vi "GV-PlotRscaleIndicator.vi"(4 "Format":string, 5 "ActualValues":dbl[](array[numeric]), 6 "type":enum16{"background", "foreground"}(ring), 7 "Graph-ref":refnum<vi>, 8 "error in (no error)":errorcluster, 9 "SelProperties":T1[](array[typedef]), 10 "Plot":i32, 11 "Picture IN":picture) -> (0 "error out":errorcluster, 3 "Picture OUT":picture)   [LabVIEW 2020, in "Sgraph_lib_V1.lvlib" / "Gviewer.lvclass"]
doc: "Andre Koelewijn, 17 feb 2022\n\nPlot an indicator on the Right side of the Graph"
uses:
  Gviewer.lvclass
  controls/Typedef_SelProperties.ctl
  controls/Typedef_LineType.ctl
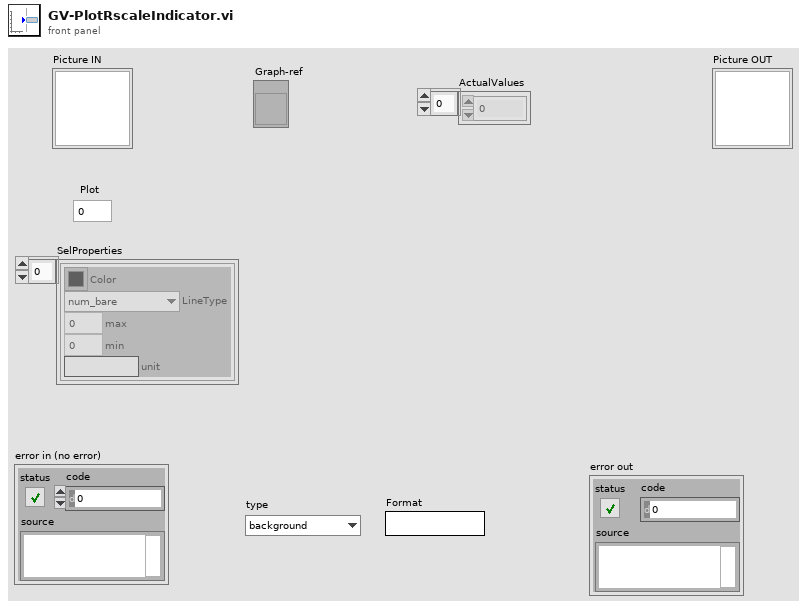
[diagram p1: front panel]
types:
  T1 = typedef "Sgraph_lib_V1.lvlib/Gviewer.lvclass/Typedef_SelProperties.ctl" = cluster{"Color":u32, "LineType":T2, "max":dbl, "min":dbl, "unit":string}
  T2 = typedef "Sgraph_lib_V1.lvlib/Gviewer.lvclass/Typedef_LineType.ctl" = enum16{"num_bare", "num_MinMax_Area", "num_MinMax_Lines", "num_MinMax_Forfor", "num_Max_Area", "num_Max_Line", "num_Max_Forfor", "num_Min_Area", "num_Min_Line", "num_Min_Fosfor", "Boolean_Line_01", "Boolean_Area_01", "Boolean_Fosfor_01", "Boolean_Line_TF", "Boolean_Area_TF", "Boolean_Fosfor_TF", "Boolean_OnOff_Line", "Boolean_OnOff_Area", "Boolean_OnOff_Fosfor", "Boolean_spare", "StringEvent_Line", "StringEvent_TimeLine"}
  T3 = cluster{"horizontal":enum16{"left", "center", "right"}, "vertical":enum16{"top", "center", "bottom"}}
  T4 = typedef "LVRectTypeDef.ctl" = cluster{"Left":i16, "Top":i16, "Right":i16, "Bottom":i16}
  T5 = typedef "LVPoint32TypeDef.ctl" = cluster{"Horizontal":i32, "Vertical":i32}
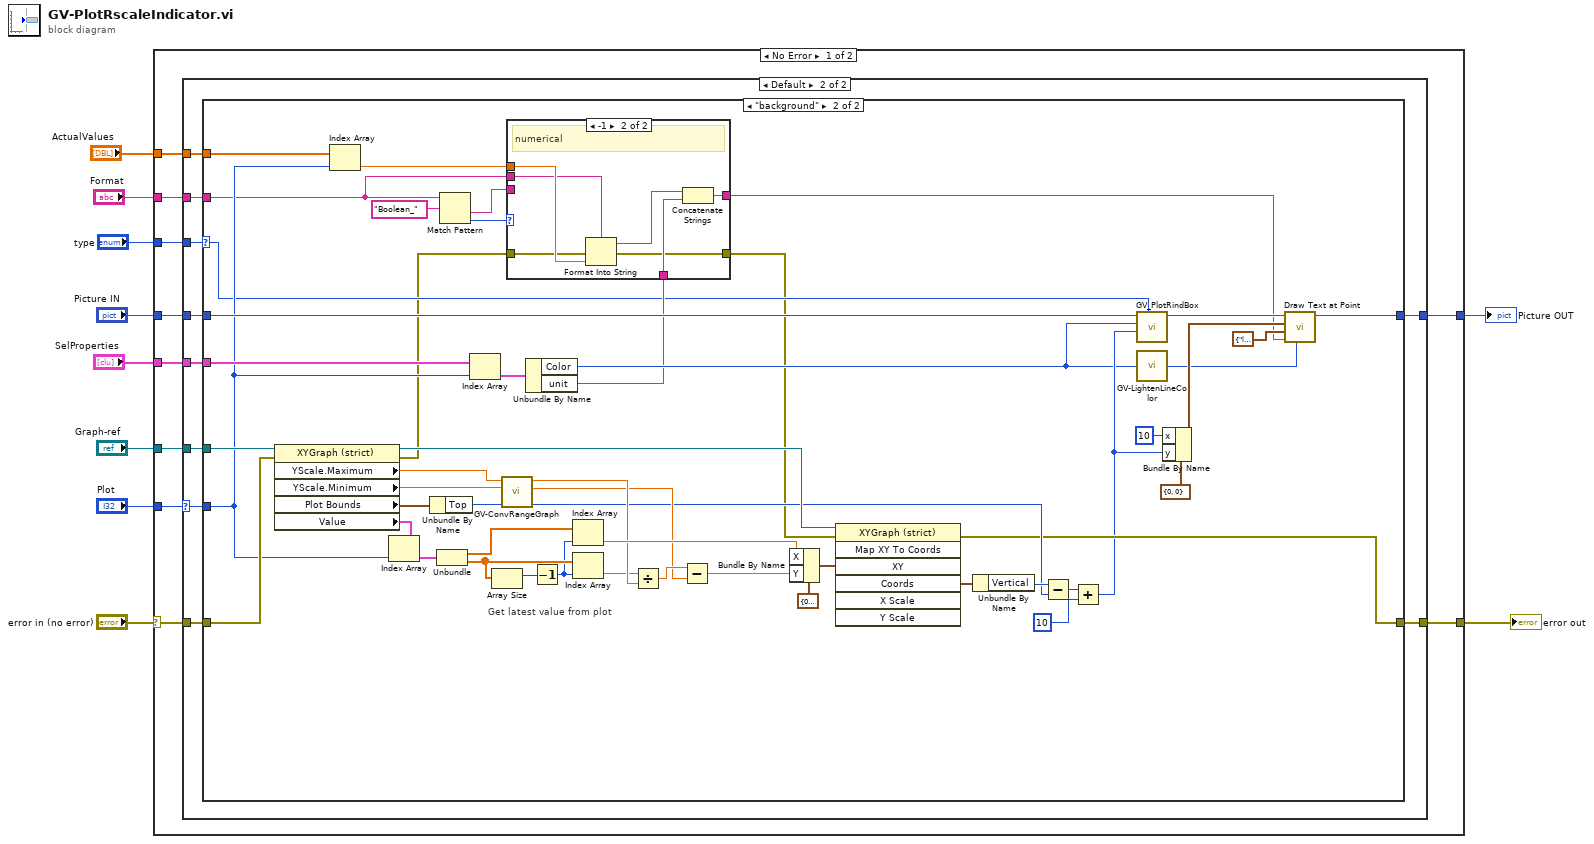
[diagram p0: block diagram]
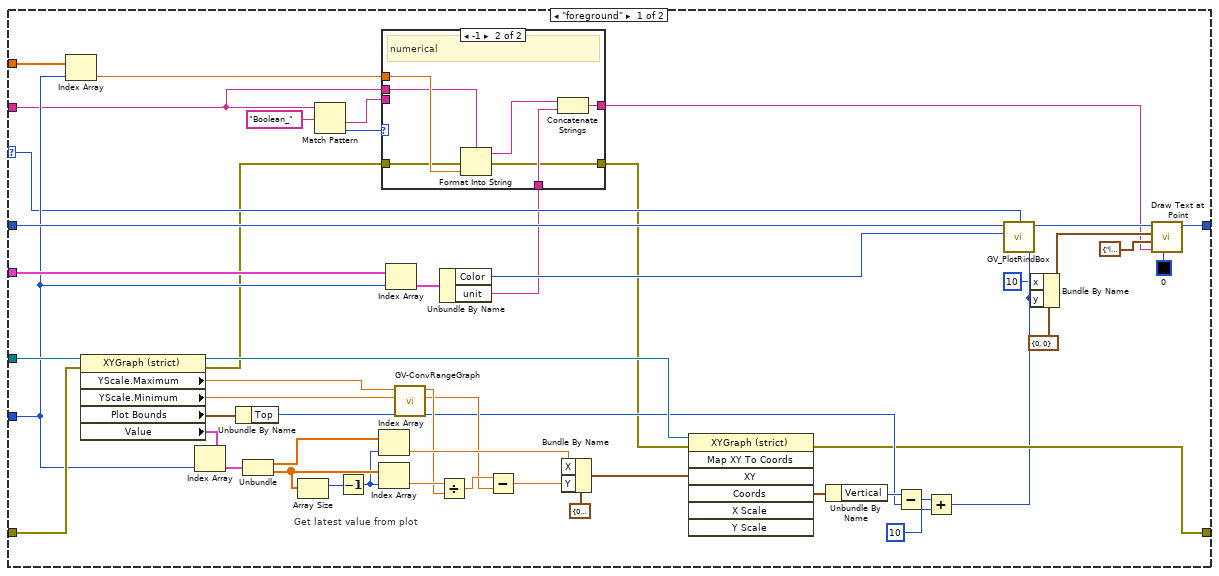
[diagram p3: hidden frame]
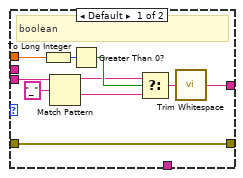
[diagram p4: hidden frame]
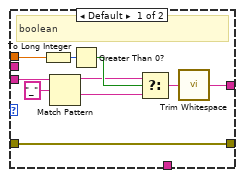
[diagram p5: hidden frame]
diagram:
  n1 = case shown="No Error" "error in (no error)" {
    selector: "error in (no error)" -> [w18 w168]
    tunnel: "Graph-ref" -> [w20 _]
    tunnel: "Plot" -> [w19 _]
    tunnel: [w17 w168] -> w7
    tunnel: "Picture IN" -> [w16 w167]
    tunnel: [w15 w167] -> w5
    tunnel: "SelProperties" -> [w14 _]
    tunnel: "type" -> [w13 _]
    tunnel: "Format" -> [w12 _]
    tunnel: "ActualValues" -> [w11 _]
    frame No Error {
      n2 = case shown="Default" w19 {
        selector: w19 -> [_ w29]
        tunnel: w20 -> [_ w32]
        tunnel: w18 -> [w22 w31]
        tunnel: [w22 w27] -> w17
        tunnel: w16 -> [w21 w28]
        tunnel: [w21 w26] -> w15
        tunnel: w14 -> [_ w30]
        tunnel: w13 -> [_ w25]
        tunnel: w12 -> [_ w24]
        tunnel: w11 -> [_ w23]
        frame -1 {
        }
        frame Default {
          n3 = case shown="\"background\"" w25 {
            selector: w25 -> [w39 w104]
            tunnel: w32 -> [w82 w149]
            tunnel: w31 -> [w80 w147]
            tunnel: w30 -> [w69 w136]
            tunnel: w29 -> [w44 w110]
            tunnel: w28 -> [w58 w126]
            tunnel: [w57 w125] -> w27
            tunnel: [w55 w123] -> w26
            tunnel: w24 -> [w33 w100]
            tunnel: w23 -> [w45 w111]
            frame "foreground" {
              # "Get latest value from plot"
              n4 = Index Array(array=w45, index=w44) -> (element=w38:dbl)
              n5 = property class="XYGraph (strict)"(reference=w82, error in=w80) -> (reference out=w72:refnum<vi>, error out=w37:errorcluster, "YScale.Maximum"=w47:dbl, "YScale.Minimum"=w46:dbl, "Plot Bounds"=w62:T4, "Value"=w63:cluster{dbl[], "data":dbl[]}[])
              n6 = Index Array(array=w63, index=w44) -> (element=w79:cluster{dbl[], "data":dbl[]})
              n7 = Unbundle By Name(w62) -> ("Top"=w61:i16)
              n8 = Unbundle(w79) -> (w74:dbl[], "data"=w78:dbl[])
              n9 = Array Size(array=w78) -> (size(s)=w81:i32)
              n10 = Match Pattern(string=w33, regular expression="Boolean_") -> (after substring=w41:string, offset past match=w42:i32)  [unwired: 1 in, 2 out]
              n11 = Decrement(x=w81) -> (x-1=w75:i32)
              n12 = Index Array(array=w74, index=w75) -> (element=w73:dbl)
              n13 = Index Array(array=w78, index=w75) -> (element=w67:dbl)
              n14 = Index Array(array=w69, index=w44) -> (element=w68:T1)
              n15 = call "GV-ConvRangeGraph.vi"("RangeL"=w46, "RangeH"=w47) -> ("Offset"=w64:dbl, "Gain"=w66:dbl)  [unwired: 8 in]
              n16 = Divide(x=w67, y=w66) -> (x/y=w65:dbl)
              n17 = Unbundle By Name(w68) -> ("Color"=w50:u32, "unit"=w35:string)
              n18 = case shown="-1" w42 {
                tunnel: w41 -> [w92 _]
                tunnel: w38 -> [w90 w99]
                tunnel: w35 -> [_ w97]
                tunnel: [w84 w96] -> w34
                tunnel: w37 -> [w83 w95]
                tunnel: [w83 w94] -> w36
                tunnel: w33 -> [_ w93]
                frame Default {
                  # "boolean"
                  n19 = To Long Integer(number=w90) -> (32bit integer=w89:i32)
                  n20 = Match Pattern(string=w92, regular expression="_") -> (before substring=w87:string, after substring=w86:string)  [unwired: 1 in, 2 out]
                  n21 = Greater Than 0?(x=w89) -> (x > 0?=w88:bool)
                  n22 = Select(t=w87, s=w88, f=w86) -> (s? t:f=w85:string)
                  n23 = call <vilib>:"Trim Whitespace.vi"("string"=w85) -> ("trimmed string"=w84:string)  [unwired: 1 in]
                }
                frame -1 {
                  # "numerical"
                  n24 = Format Into String(format string=w93, error in=w95, w99) -> (resulting string=w98:string, error out=w94:errorcluster)  [unwired: 1 in]
                  n25 = Concatenate Strings(w98, w97) -> (w96:string)
                }
              }
              n26 = Subtract(x=w65, y=w64) -> (x-y=w43:dbl)
              n27 = Bundle By Name(cluster=cluster{"X":dbl, "Y":dbl} {"X"=0.0, "Y"=0.0} ("XY"), "X"=w73, "Y"=w43) -> (w76:cluster{"X":dbl, "Y":dbl})
              n28 = invoke class="XYGraph (strict)" method="Map XY To Coords"(reference=w72, error in=w36, "XY"=w76) -> (error out=w57:errorcluster, "Coords"=w71:T5)  [unwired: 4 in, 5 out]
              n29 = Unbundle By Name(w71) -> ("Vertical"=w70:i32)
              n30 = Subtract(x=w70, y=w61) -> (x-y=w60:i32)
              n31 = Add(x=w60, y=10) -> (x+y=w53:i32)
              n32 = call "GV_PlotRindBox.vi"("type"=w39, "Vertical"=w53, "color(black)"=w50, "Picture IN"=w58) -> ("Picture OUT"=w56:picture)  [unwired: 7 in]
              n33 = Bundle By Name(cluster=cluster{"x":i16, "y":i16} {"x"=0, "y"=0} ("origin"), "x"=i16 10, "y"=w53) -> (w51:cluster{"x":i16, "y":i16})
              n34 = call <vilib>:"Draw Text at Point.vi"("text color(black)"=u32 0, "text"=w34, "alignment(left, top)"=T3 {"horizontal"=enum."left", "vertical"=enum."center"}, "origin"=w51, "picture"=w56) -> ("new picture"=w55:picture)  [unwired: 5 in, 1 out]
            }
            frame "background" {
              # "Get latest value from plot"
              n35 = property class="XYGraph (strict)"(reference=w149, error in=w147) -> (reference out=w139:refnum<vi>, error out=w103:errorcluster, "YScale.Maximum"=w115:dbl, "YScale.Minimum"=w114:dbl, "Plot Bounds"=w130:T4, "Value"=w131:cluster{dbl[], "data":dbl[]}[])
              n36 = Index Array(array=w111, index=w110) -> (element=w106:dbl)
              n37 = Index Array(array=w131, index=w110) -> (element=w146:cluster{dbl[], "data":dbl[]})
              n38 = Unbundle By Name(w130) -> ("Top"=w129:i16)
              n39 = Unbundle(w146) -> (w141:dbl[], "data"=w145:dbl[])
              n40 = Match Pattern(string=w100, regular expression="Boolean_") -> (after substring=w107:string, offset past match=w108:i32)  [unwired: 1 in, 2 out]
              n41 = Index Array(array=w136, index=w110) -> (element=w135:T1)
              n42 = Array Size(array=w145) -> (size(s)=w148:i32)
              n43 = call "GV-ConvRangeGraph.vi"("RangeL"=w114, "RangeH"=w115) -> ("Offset"=w132:dbl, "Gain"=w134:dbl)  [unwired: 8 in]
              n44 = Unbundle By Name(w135) -> ("Color"=w118:u32, "unit"=w105:string)
              n45 = case shown="-1" w108 {
                tunnel: w107 -> [w159 _]
                tunnel: w106 -> [w157 w166]
                tunnel: w105 -> [_ w164]
                tunnel: [w151 w163] -> w101
                tunnel: w103 -> [w150 w162]
                tunnel: [w150 w161] -> w102
                tunnel: w100 -> [_ w160]
                frame Default {
                  # "boolean"
                  n46 = To Long Integer(number=w157) -> (32bit integer=w156:i32)
                  n47 = Match Pattern(string=w159, regular expression="_") -> (before substring=w154:string, after substring=w153:string)  [unwired: 1 in, 2 out]
                  n48 = Greater Than 0?(x=w156) -> (x > 0?=w155:bool)
                  n49 = Select(t=w154, s=w155, f=w153) -> (s? t:f=w152:string)
                  n50 = call <vilib>:"Trim Whitespace.vi"("string"=w152) -> ("trimmed string"=w151:string)  [unwired: 1 in]
                }
                frame -1 {
                  # "numerical"
                  n51 = Format Into String(format string=w160, error in=w162, w166) -> (resulting string=w165:string, error out=w161:errorcluster)  [unwired: 1 in]
                  n52 = Concatenate Strings(w165, w164) -> (w163:string)
                }
              }
              n53 = Decrement(x=w148) -> (x-1=w142:i32)
              n54 = Index Array(array=w141, index=w142) -> (element=w140:dbl)
              n55 = Index Array(array=w145, index=w142) -> (element=w113:dbl)
              n56 = Divide(x=w113, y=w134) -> (x/y=w133:dbl)
              n57 = Subtract(x=w133, y=w132) -> (x-y=w112:dbl)
              n58 = Bundle By Name(cluster=cluster{"X":dbl, "Y":dbl} {"X"=0.0, "Y"=0.0} ("XY"), "X"=w140, "Y"=w112) -> (w143:cluster{"X":dbl, "Y":dbl})
              n59 = invoke class="XYGraph (strict)" method="Map XY To Coords"(reference=w139, error in=w102, "XY"=w143) -> (error out=w125:errorcluster, "Coords"=w138:T5)  [unwired: 4 in, 5 out]
              n60 = Unbundle By Name(w138) -> ("Vertical"=w137:i32)
              n61 = Subtract(x=w137, y=w129) -> (x-y=w128:i32)
              n62 = Add(x=w128, y=10) -> (x+y=w121:i32)
              n63 = call "GV_PlotRindBox.vi"("type"=w104, "Vertical"=w121, "color(black)"=w118, "Picture IN"=w126) -> ("Picture OUT"=w124:picture)  [unwired: 7 in]
              n64 = call "GV-LightenLineColor.vi"("Line color"=w118) -> ("Light color"=w117:u32)  [unwired: 6 in]
              n65 = Bundle By Name(cluster=cluster{"x":i16, "y":i16} {"x"=0, "y"=0} ("origin"), "x"=i16 10, "y"=w121) -> (w119:cluster{"x":i16, "y":i16})
              n66 = call <vilib>:"Draw Text at Point.vi"("text color(black)"=w117, "text"=w101, "alignment(left, top)"=T3 {"horizontal"=enum."left", "vertical"=enum."center"}, "origin"=w119, "picture"=w124) -> ("new picture"=w123:picture)  [unwired: 5 in, 1 out]
            }
          }
        }
      }
    }
    frame Error {
    }
  }
  "Picture OUT" <- w5
  "error out" <- w7
